vi "Waveform Gap.vi"(8 "error in":errorcluster, 10 "Current Block":waveform(sgl)[](array[waveform]), 11 "DAQ Actor in":refnum<class "DAQ Actor.lvclass">) -> (0 "error out":errorcluster, 1 "Output Block":bool, 2 "Gapped Wfm Data":waveform(sgl)[](array[waveform]), 3 "DAQ Actor out":refnum<class "DAQ Actor.lvclass">)   [LabVIEW 2012, in "Data Acquisition.lvlib" / "DAQ Actor.lvclass"]
uses:
  DAQ Actor.lvclass
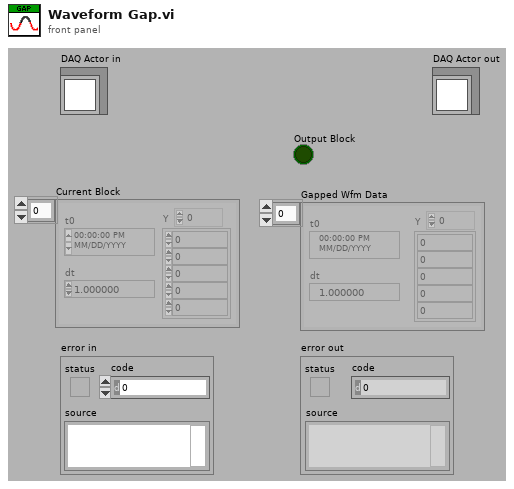
[diagram p1: front panel]
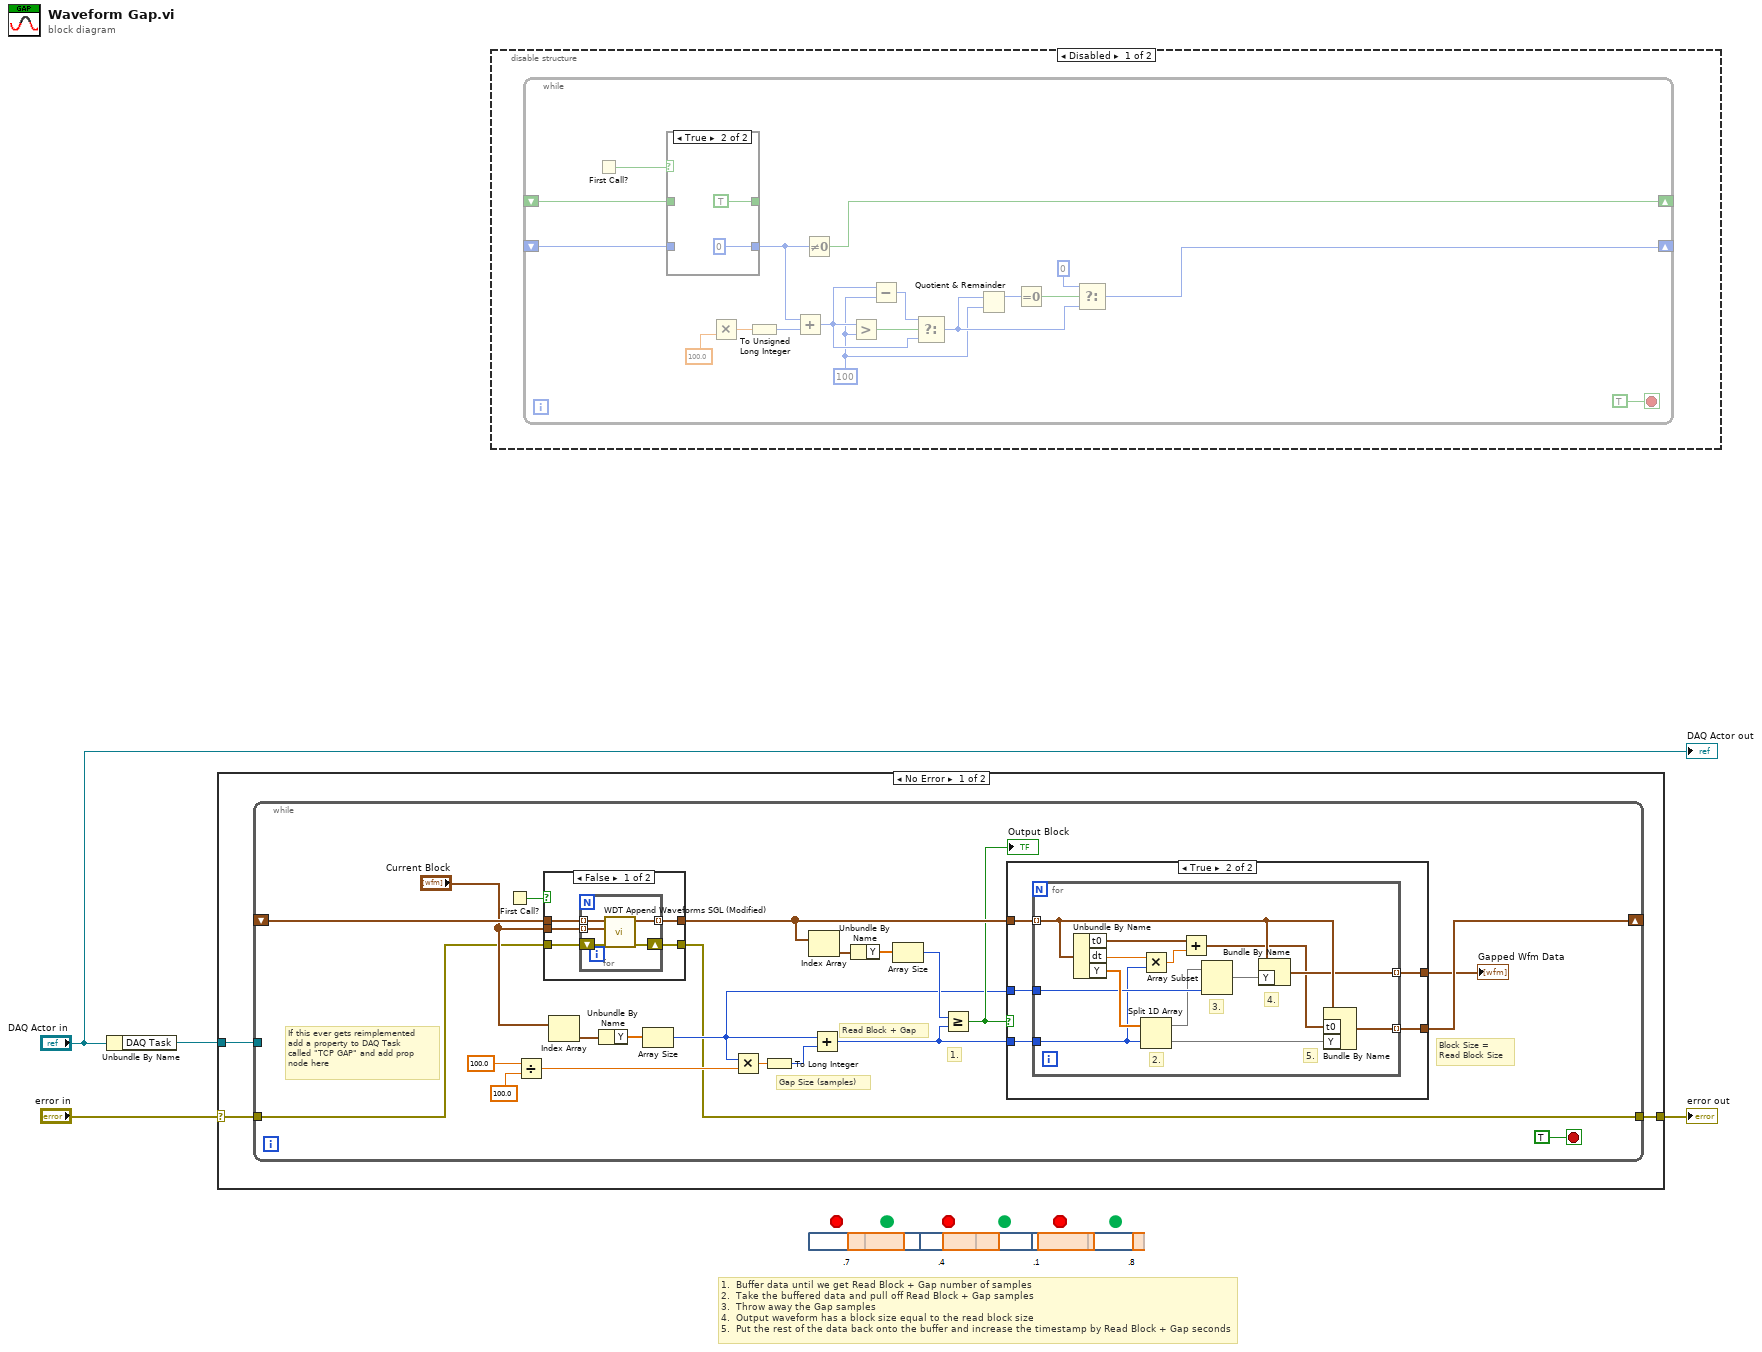
[diagram p0: block diagram]
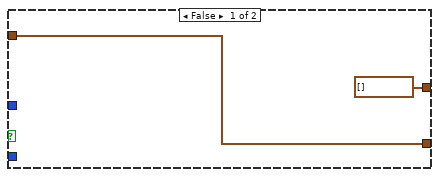
[diagram p2: hidden frame]
diagram:
  # "1.  Buffer data until we get Read Block + Gap number of samples\n2.  Take the buffered data and pull off Read Block + Gap samples\n3.  Throw away the Gap samples\n4.  Output waveform has a block size equal to the read block size\n5.  Put the rest of the data back onto the buffer and increase the timestamp by Read Block + Gap seconds"
  n1 = Unbundle By Name("DAQ Actor in") -> ("DAQ Task"=w1:refnum<class "DAQ Task.lvclass">)
  n2 = case shown="No Error" "error in" {
    selector: "error in" -> [w7 w62]
    tunnel: [w6 w62] -> w4
    tunnel: w1 -> [w5 _]
    frame No Error {
      n3 = while {
        shift-right: [w15] -> _
        shift-left: _ -> [w19]
        tunnel: w7 -> [w9]
        tunnel: [w11] -> w6
        tunnel: w5 -> [_]
        stop <- TRUE stop-if-true
        # "If this ever gets reimplemented\nadd a property to DAQ Task\ncalled \"TCP GAP\" and add prop\nnode here"
        # "Read Block + Gap"
        # "1."
        # "Block Size = \nRead Block Size"
        # "Gap Size (samples)"
        n4 = First Call?() -> (First Call?: T/F=w28:bool)
        n5 = Divide(x=100.0, y=100.0) -> (x/y=w24:dbl)
        n6 = case shown="False" w28 {
          tunnel: w19 -> [w54 _]
          tunnel: "Current Block" -> [w53 w60]
          tunnel: [w50 w60] -> w18
          tunnel: w9 -> [w52 w61]
          tunnel: [w51 w61] -> w11
          frame False {
            n7 = for {
              tunnel: w53 -> [w59] mode=indexing
              tunnel: w54 -> [w58] mode=indexing
              tunnel: [w57] -> w50 mode=indexing
              shift-right: [w55] -> w51
              shift-left: w52 -> [w56]
              n8 = call "WDT Append Waveforms SGL (Modified).vi"("error in (no error)"=w56, "waveform B"=w59, "waveform A"=w58) -> ("error out"=w55:errorcluster, "waveform out"=w57:waveform(sgl))  [unwired: 7 in]
            }
          }
          frame True {
          }
        }
        n9 = Index Array(array="Current Block") -> (element=w27:waveform(sgl))  [unwired: 1 in]
        n10 = Unbundle By Name(w27) -> ("Y"=w26:sgl[])
        n11 = Array Size(array=w26) -> (size(s)=w13:i32)
        n12 = Multiply(x=w13, y=w24) -> (x*y=w23:dbl)
        n13 = To Long Integer(number=w23) -> (32bit integer=w22:i32)
        n14 = Index Array(array=w18) -> (element=w21:waveform(sgl))  [unwired: 1 in]
        n15 = Add(x=w13, y=w22) -> (x+y=w17:i32)
        n16 = Unbundle By Name(w21) -> ("Y"=w20:sgl[])
        n17 = Array Size(array=w20) -> (size(s)=w16:i32)
        n18 = Greater Or Equal?(x=w16, y=w17) -> (x >= y?=w14:bool)
        "Output Block" <- w14
        n19 = case shown="True" w14 {
          tunnel: w18 -> [w31 w36]
          tunnel: w17 -> [_ w35]
          tunnel: [w31 w34] -> w15
          tunnel: [waveform(sgl)[] [] w33] -> w10
          tunnel: w13 -> [_ w32]
          frame False {
          }
          frame True {
            n20 = for {
              tunnel: w36 -> [w46] mode=indexing
              tunnel: w35 -> [w42]
              tunnel: w32 -> [w48]
              tunnel: [w45] -> w34 mode=indexing
              tunnel: [w44] -> w33 mode=indexing
              # "5."
              # "4."
              # "3."
              # "2."
              n21 = Unbundle By Name(w46) -> ("t0"=w40:timestamp, "dt"=w43:dbl, "Y"=w49:sgl[])
              n22 = Multiply(x=w43, y=w42) -> (x*y=w41:dbl)
              n23 = Split 1D Array(array=w49, index=w42) -> (first subarray=w38:sgl[], second subarray=w47:sgl[])
              n24 = Add(x=w40, y=w41) -> (x+y=w39:timestamp)
              n25 = Array Subset(array=w38, length=w48) -> (w37:sgl[])  [unwired: 1 in]
              n26 = Bundle By Name(cluster=w46, "Y"=w37) -> (w44:waveform(sgl))
              n27 = Bundle By Name(cluster=w46, "t0"=w39, "Y"=w47) -> (w45:waveform(sgl))
            }
          }
        }
        "Gapped Wfm Data" <- w10
      }
    }
    frame Error {
    }
  }
  "error out" <- w4
  n28 = disable-structure shown="Disabled" {
    frame Disabled {
      n29 = while {
        shift-right: [w80] -> _
        shift-left: _ -> [w79]
        shift-right: [w75] -> _
        shift-left: _ -> [w74]
        stop <- TRUE stop-if-true
        w63 = u32 100 ("y")
        n30 = First Call?() -> (First Call?: T/F=w81:bool)
        n31 = case shown="True" w81 {
          tunnel: [w83 u32 0 ("Interval Pos")] -> w77
          tunnel: w79 -> [w83 _]
          tunnel: [w82 TRUE ("Output Block")] -> w76
          tunnel: w74 -> [w82 _]
          frame False {
          }
          frame True {
          }
        }
        n32 = Multiply(y=100.0) -> (x*y=w70:dbl)  [unwired: 1 in]
        n33 = To Unsigned Long Integer(number=w70) -> (unsigned 32bit integer=w71:u32)
        n34 = Add(x=w77, y=w71) -> (x+y=w65:u32)
        n35 = Not Equal To 0?(x=w77) -> (x != 0?=w75:bool)
        n36 = Greater?(x=w65, y=w63) -> (0:w67:bool)
        n37 = Subtract(x=w65, y=w63) -> (x-y=w66:u32)
        n38 = Select(t=w66, s=w67, f=w65) -> (s? t:f=w64:u32)
        n39 = Quotient & Remainder(x=w64, y=w63) -> (x-y*floor(x/y)=w69:u32)  [unwired: 1 out]
        n40 = Equal To 0?(x=w69) -> (x = 0?=w68:bool)
        n41 = Select(t=u32 0, s=w68, f=w64) -> (s? t:f=w80:u32)
      }
    }
    frame Enabled {
    }
  }
  "DAQ Actor out" <- "DAQ Actor in"
